vi "HistogramManual1001.vi"   [LabVIEW 2013]
uses:
  <vilib>/Heliosphere Research LLC/Advanced Plotting Toolkit/api_plotting/Histogram_Manual.vi
  <vilib>/Heliosphere Research LLC/Advanced Plotting Toolkit/Advanced Plotting Toolkit.lvlib
types:
  T1 = typedef "Advanced Plotting Toolkit.lvlib/PlotID.ctl" = i32
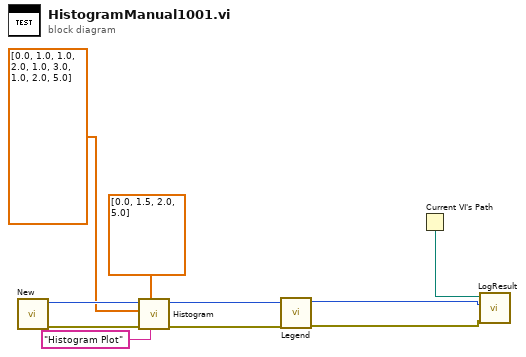
[diagram p0: block diagram]
diagram:
  n1 = call <vilib>:"New.vi"() -> ("error out"=w8:errorcluster, "Plot ID"=w10:T1)  [unwired: 10 in]
  n2 = call-poly <vilib>:"Histogram.vi"("Legend Title"="Histogram Plot", "Bins"=dbl[] [0.0, 1.5, 2.0, 5.0], "error in (no error)"=w8, "Data"=dbl[] [0.0, 1.0, 1.0, 2.0, 1.0, 3.0, 1.0, 2.0, 5.0], "Plot ID"=w10) -> ("error out"=w3:errorcluster, "Plot ID Out"=w5:T1)  [unwired: 5 in]
  n3 = call <vilib>:"Legend.vi"("error in (no error)"=w3, "Plot ID"=w5) -> ("error out"=w2:errorcluster, "Plot ID Out"=w4:T1)  [unwired: 8 in]
  n4 = Current VI's Path() -> (path=w9:path)
  n5 = call "LogResult.vi"("Test Result"=w2, "Test Artifact"=w4, "VI Path"=w9) -> ()  [unwired: 9 in]
